vi "SetNeoPixelBuf.vi"(8 "error in (no error)":errorcluster, 9 "Color Box":u32(colorbox), 10 "Address":u16, 11 "AdaFruit-Seesaw in":refnum<class "AdaFruit-Seesaw.lvclass">) -> (0 "error out":errorcluster, 3 "AdaFruit-Seesaw out":refnum<class "AdaFruit-Seesaw.lvclass">)   [LabVIEW 2020, in "CTI-Peripheral.lvlib" / "AdaFruit-Seesaw.lvclass"]
uses:
  AdaFruit-Seesaw.lvclass
  Private/SeeSawBaseAddresses.ctl
  Private/SeeSawNEOPIXELFunctions.ctl
  AdaFruit-Seesaw.lvclass/AdaFruit-Seesaw.ctl
  CTI/I2C Connection/I2C Connection.lvclass/I2C Connection.ctl
  CTI/Session/I2C Write Data.vi
  CTI/I2C Connection/I2C Connection.lvclass
panel:
  out "string":string
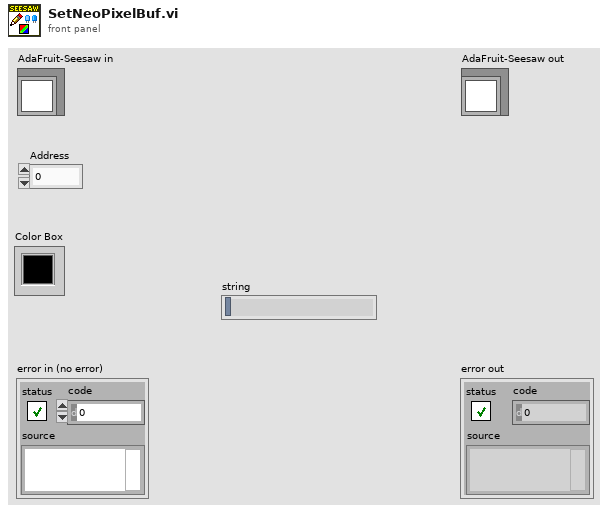
[diagram p1: front panel]
types:
  T1 = typedef "CTI-Peripheral.lvlib/AdaFruit-Seesaw.lvclass/SeeSawNEOPIXELFunctions.ctl" = u8
  T2 = typedef "CTI-Peripheral.lvlib/AdaFruit-Seesaw.lvclass/SeeSawBaseAddresses.ctl" = u8
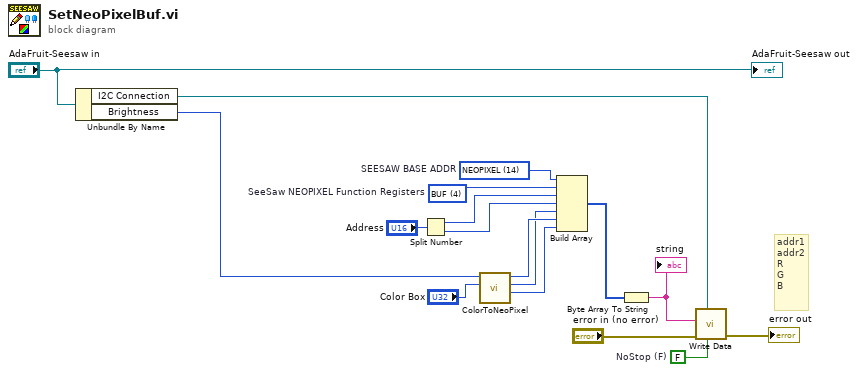
[diagram p0: block diagram]
diagram:
  w10 = T1 4 items=["STATUS", "PIN", "SPEED", "BUF_LENGTH", "BUF", "SHOW"]  # SeeSaw NEOPIXEL Function Registers
  w15 = FALSE  # NoStop (F)
  w17 = T2 14 items=["STATUS"=0, "GPIO"=1, "SERCOM0"=2, "TIMER"=8, "ADC"=9, "DAC"=10, "INTERUPT"=11, "DAP"=12, "EEPROM"=13, "NEOPIXEL"=14, "TOUCH"=15, "KEYPAD"=16, "ENCODER"=17, "SPECTRUM"=18]  # SEESAW BASE ADDR
  # "addr1\naddr2\nR\nG\nB"
  n1 = Unbundle By Name("AdaFruit-Seesaw in") -> ("I2C Connection"=w16:refnum<class "I2C Connection.lvclass">, "Brightness"=w1:u8)
  n2 = Split Number(x="Address") -> (hi(x)=w8:u8, lo(x)=w7:u8)
  n3 = call "ColorToNeoPixel.vi"("Color Box"="Color Box", "Lightness"=w1) -> ("NeoPBlue"=w6:u8, "NeoPGreen"=w2:u8, "NeoPRed"=w3:u8)  [unwired: 7 in]
  n4 = Build Array(w17, w10, w8, w7, w2, w3, w6) -> (w4:T1[])
  n5 = Byte Array To String(unsigned byte array=w4) -> (string=w14:string)
  "string" <- w14
  n6 = call "Write Data.vi"("NoStop (F)"=w15, "I2C Connection"=w16, "error in (no error)"="error in (no error)", "Data"=w14) -> ("error out"=→"error out":errorcluster)  [unwired: 7 in]
  "AdaFruit-Seesaw out" <- "AdaFruit-Seesaw in"
